vi "Gerakan Sekuensial.vi"() -> ()   [LabVIEW 2011]
uses:
  <vilib>/Instr/_visa.llb/VISA Configure Serial Port (Instr).vi
panel:
  in  "Numeric":i32
  in  "write buffer":string
  out "Result":string
  in  "STOP":bool
  in  "VISA resource name":refnum<visa-resource-name>="COM1"
  in  "Time":dbl=500.0
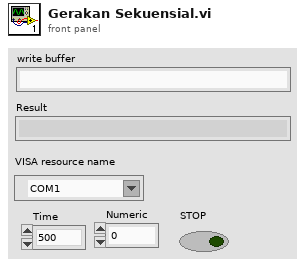
[diagram p1: front panel]
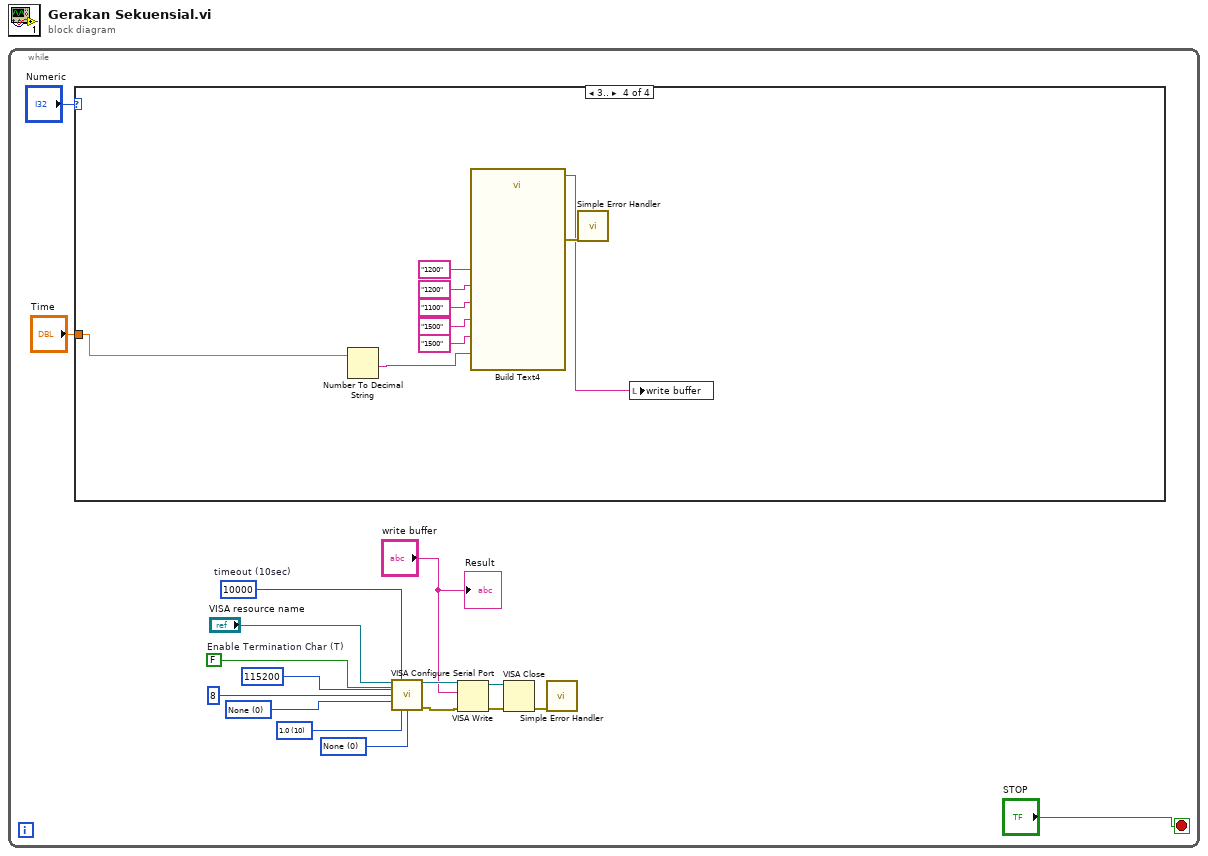
[diagram p0: block diagram]
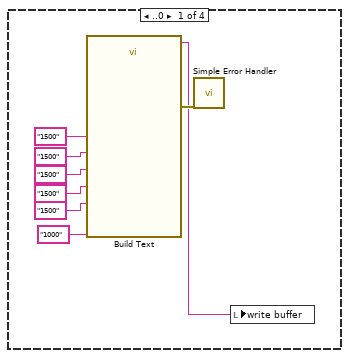
[diagram p2: hidden frame]
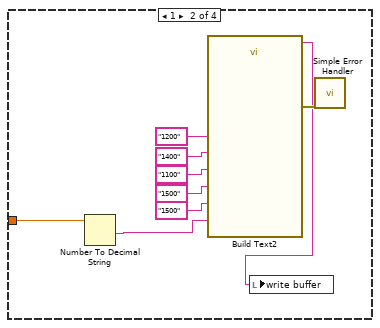
[diagram p3: hidden frame]
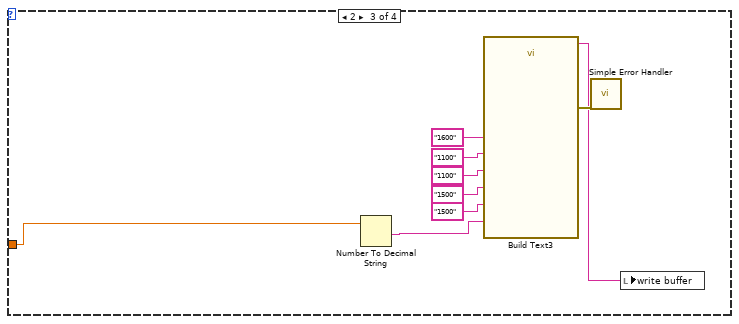
[diagram p4: hidden frame]
diagram:
  n1 = while {
    stop <- "STOP" stop-if-true
    w11 = u16 0 items=["None"=0, "XON/XOFF"=1, "RTS/CTS"=2, "DTR/DSR"=4] ("flow control")
    w12 = u16 10 items=["1.0"=10, "1.5"=15, "2.0"=20] ("stop bits")
    w15 = u16 0 items=["None", "Odd", "Even", "Mark", "Space"] ("parity")
    w13 = FALSE  # Enable Termination Char (T)
    w14 = u32 10000  # timeout (10sec)
    n2 = case shown="3.." "Numeric" {
      tunnel: "Time" -> [_ w26 w35 w44]
      frame ..0 {
        n3 = call "Build Text"("pwm3"="1500", "time"="1000", "pwm0"="1500", "pwm1"="1500", "pwm2"="1500", "pwm4"="1500") -> ("Result"=w18:string, "error out"=w25:errorcluster)  [unwired: 8 in]
        n4 = call <vilib>:"Simple Error Handler.vi"("error in (no error)"=w25) -> ()  [unwired: 4 in, 5 out]
        n5 = local write "write buffer"(w18) -> ()
      }
      frame 1 {
        n6 = Number To Decimal String(number=w26) -> (decimal integer string=w34:string)  [unwired: 1 in]
        n7 = call "Build Text2"("pwm3"="1500", "time"=w34, "pwm0"="1200", "pwm1"="1400", "pwm2"="1100", "pwm4"="1500") -> ("Result"=w27:string, "error out"=w33:errorcluster)  [unwired: 8 in]
        n8 = local write "write buffer"(w27) -> ()
        n9 = call <vilib>:"Simple Error Handler.vi"("error in (no error)"=w33) -> ()  [unwired: 4 in, 5 out]
      }
      frame 2 {
        n10 = Number To Decimal String(number=w35) -> (decimal integer string=w43:string)  [unwired: 1 in]
        n11 = call "Build Text3"("pwm3"="1500", "time"=w43, "pwm0"="1600", "pwm1"="1100", "pwm2"="1100", "pwm4"="1500") -> ("Result"=w36:string, "error out"=w42:errorcluster)  [unwired: 8 in]
        n12 = call <vilib>:"Simple Error Handler.vi"("error in (no error)"=w42) -> ()  [unwired: 4 in, 5 out]
        n13 = local write "write buffer"(w36) -> ()
      }
      frame 3.. {
        n14 = Number To Decimal String(number=w44) -> (decimal integer string=w52:string)  [unwired: 1 in]
        n15 = call "Build Text4"("pwm3"="1500", "time"=w52, "pwm0"="1200", "pwm1"="1200", "pwm2"="1100", "pwm4"="1500") -> ("Result"=w45:string, "error out"=w51:errorcluster)  [unwired: 8 in]
        n16 = call <vilib>:"Simple Error Handler.vi"("error in (no error)"=w51) -> ()  [unwired: 4 in, 5 out]
        n17 = local write "write buffer"(w45) -> ()
      }
    }
    n18 = call-poly "VISA Configure Serial Port"("VISA resource name"="VISA resource name", "timeout (10sec)"=w14, "Enable Termination\nChar (T)"=w13, "baud rate (9600)"=u32 115200 ("baud rate"), "data bits (8)"=u16 8 ("data bits"), "parity (0:none)"=w15, "stop bits (10: 1 bit)"=w12, "flow control (0:none)"=w11) -> ("VISA resource name out"=w5:refnum<visa-resource-name>, "error out"=w4:errorcluster)  [unwired: 6 in]
    n19 = VISA Write(VISA resource name=w5, write buffer="write buffer", error in (no error)=w4) -> (VISA resource name out=w7:refnum<visa-resource-name>, error out=w6:errorcluster)  [unwired: 1 out]
    n20 = VISA Close(VISA resource name=w7, error in (no error)=w6) -> (error out=w8:errorcluster)
    n21 = call <vilib>:"Simple Error Handler.vi"("error in (no error)"=w8) -> ()  [unwired: 4 in, 5 out]
    "Result" <- "write buffer"
  }
